vi "Single-Line To CSM Parts.vi"(11 "Single-line Text":string="asdfas @ * >> asdfas @ asvas ->    <register> //asdfas") -> (0 "Msg Type":T4, 1 "Comment Pos":i32, 2 "Comments":T3, 3 "Property":T1[](array[typedef]))   [LabVIEW 2017]
uses:
  Single-Line Type.ctl
  CSM Part Property.ctl
  Single-Line Selection Type.ctl
  <vilib>/regexp/Match Regular Expression.xnode
  _Shared/CSM Shared.lvlib
panel:
  out "Array":string[](array[string])=["status@asdfasf ", ">>", " abcdef@xaef ", "->", "<register>"]
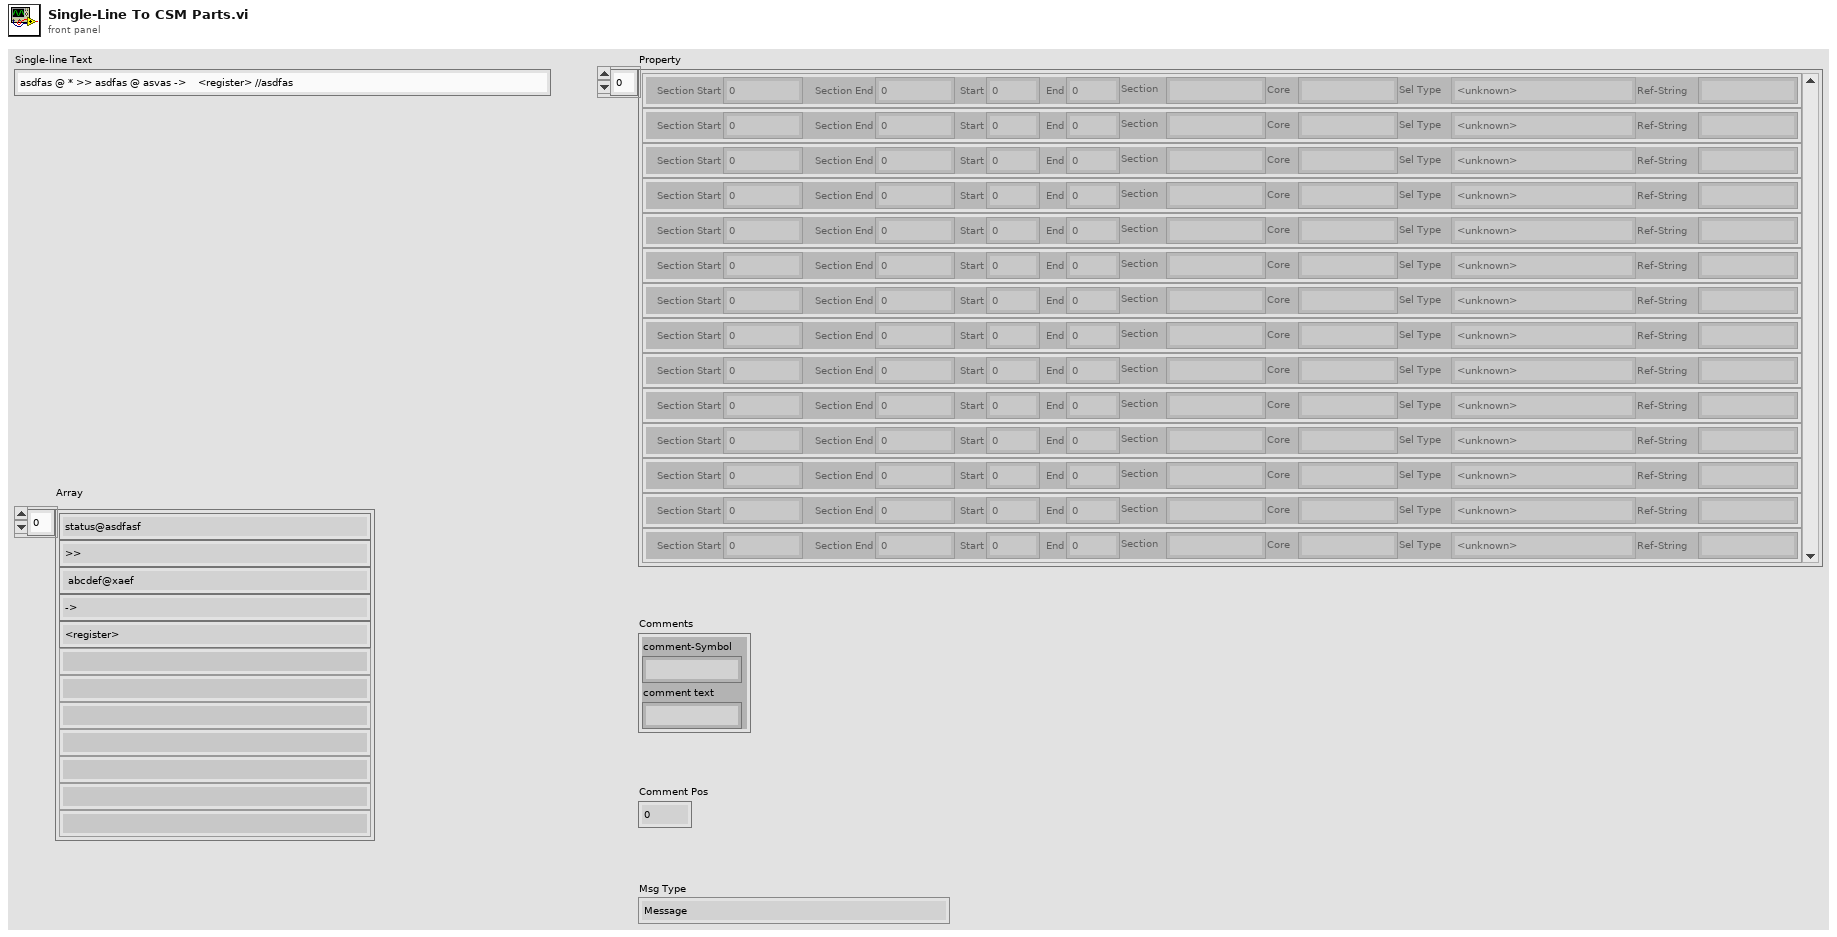
[diagram p1: front panel]
types:
  T1 = typedef "CSM Part Property.ctl" = cluster{"Section Start":u32, "Section End":u32, "Start":u32, "End":u32, "Section":string, "Core":string, "Sel Type":T2, "Ref-String":string}
  T2 = typedef "Single-Line Selection Type.ctl" = enum16{"<unknown>", "Reg-SourceSignal", "Reg-@Seperator", "Reg-ArgSymbol", "Reg-TargetAPI", "Reg-Module", "Reg-Symbol", "Reg-Oper", "Msg-State", "Msg-Arg", "Msg-ArgSymbol", "Msg-Symbol", "Msg-Module", "Broadcast-Signal", "Broadcast-ArgSymbol", "Broadcast-Arg", "Broadcast-Symbol", "Broadcast-Oper", "Comment-Symbol", "Comment-Content"}
  T3 = cluster{"comment-Symbol":string, "comment text":string}
  T4 = typedef "Single-Line Type.ctl" = enum16{"Message", "Broadcast", "Registration"}
  T5 = cluster{"Single-line Text":string, "Single-line Text":string}
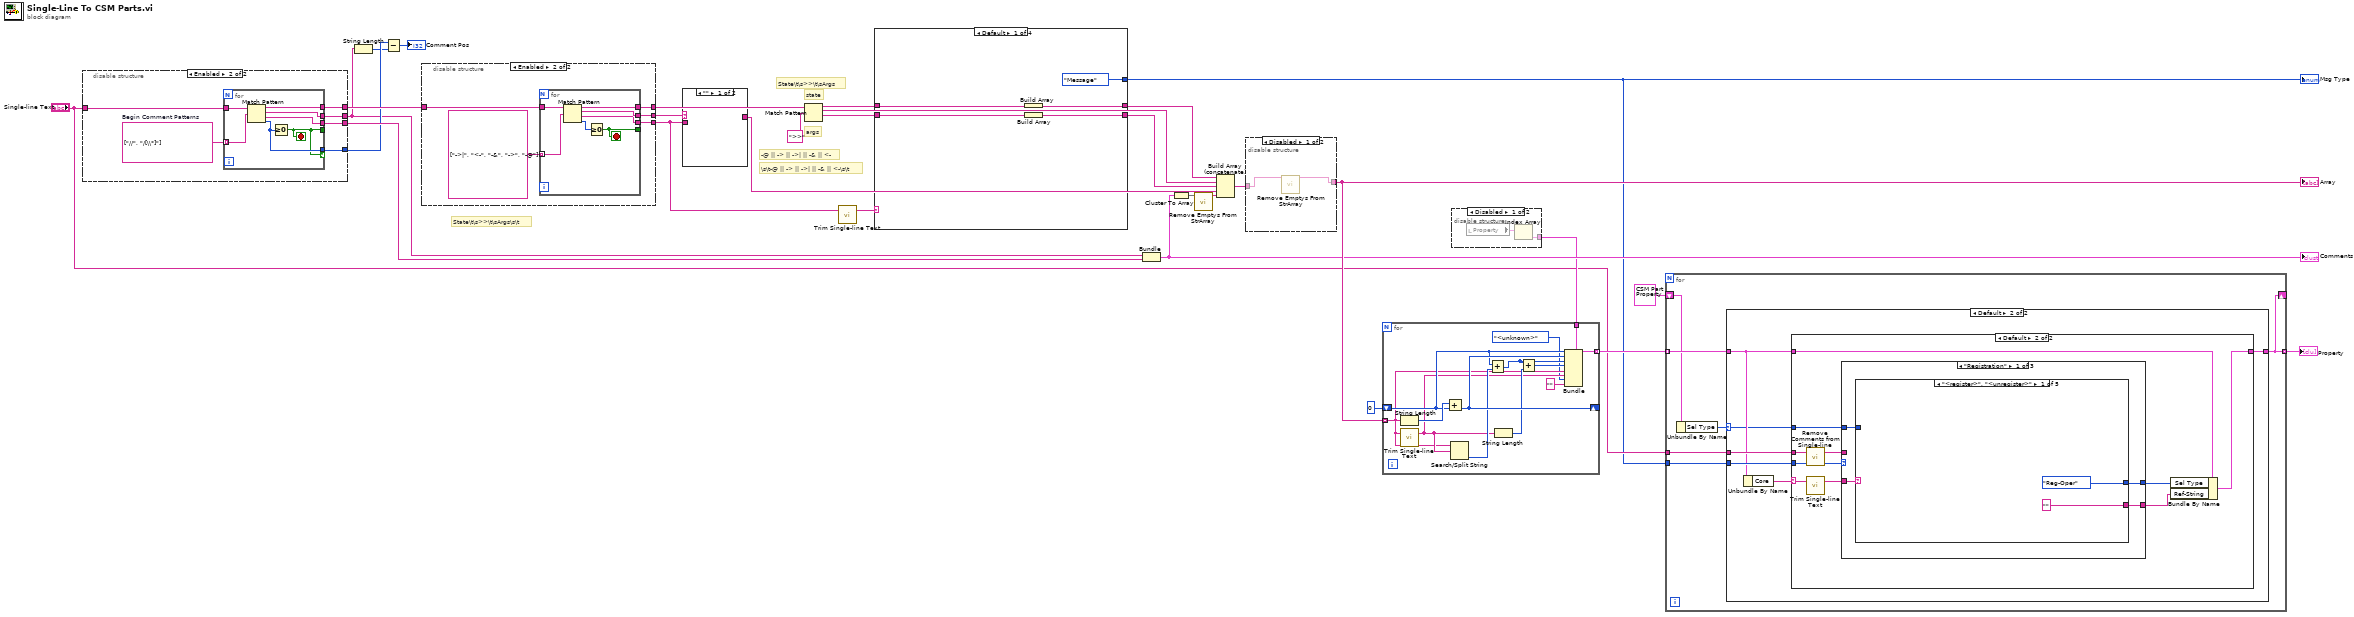
[diagram p0: block diagram]
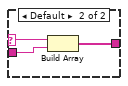
[diagram p2: hidden frame]
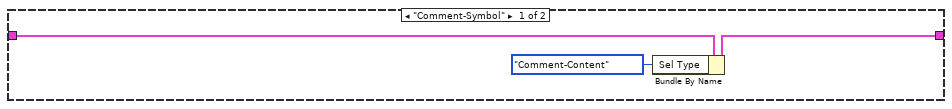
[diagram p5: hidden frame]
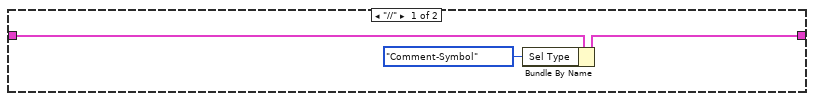
[diagram p6: hidden frame]
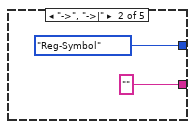
[diagram p7: hidden frame]
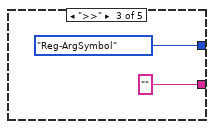
[diagram p8: hidden frame]
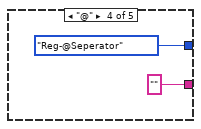
[diagram p9: hidden frame]
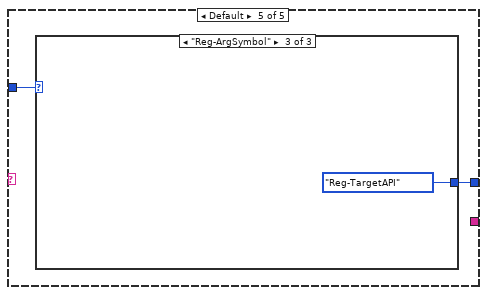
[diagram p10: hidden frame]
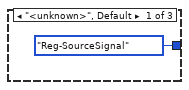
[diagram p11: hidden frame]
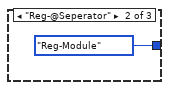
[diagram p12: hidden frame]
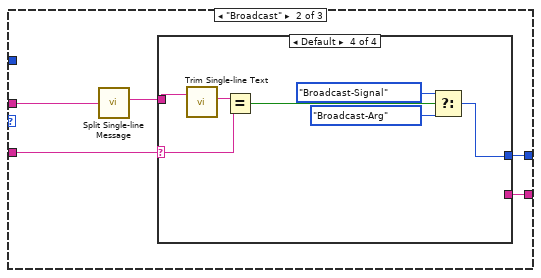
[diagram p13: hidden frame]
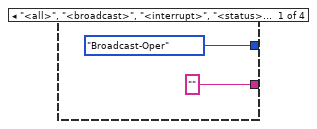
[diagram p14: hidden frame]
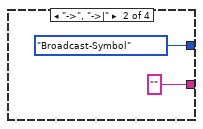
[diagram p15: hidden frame]
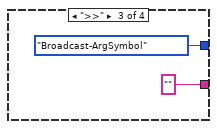
[diagram p16: hidden frame]
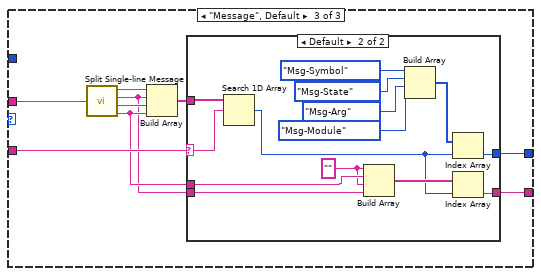
[diagram p17: hidden frame]
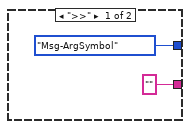
[diagram p18: hidden frame]
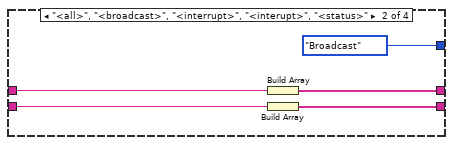
[diagram p19: hidden frame]
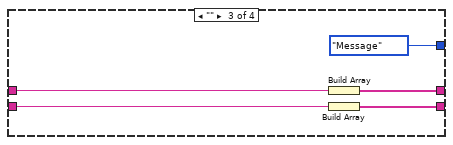
[diagram p20: hidden frame]
diagram:
  # "-@ || -> || ->| || -& || <-"
  # "\\s\\t-@ || -> || ->| || -& || <-\\s\\t"
  # "State\\t\\s>>\\t\\sArgs"
  # "State\\t\\s>>\\t\\sArgs\\s\\t"
  # "args"
  # "state"
  n1 = disable-structure shown="Enabled" {
    disable-tunnel: [w33 w153] -> w29
    disable-tunnel: [w32 w152] -> w13
    disable-tunnel: [w31 w151] -> w20
    disable-tunnel: "Single-line Text" -> [w30 w154]
    disable-tunnel: [_ w149] -> w15
    frame Disabled {
      n2 = xnode "Match Regular Expression"("input string"=w30, "regular expression"="[\\t\\s]*-@|->|<-|-&[\\t\\s]*") -> ("before match"=w33:string, "whole match"=w32:string, "after match"=w31:string)  [unwired: 4 in, 2 out]
    }
    frame Enabled {
      w150 = string[] ["//", "/[\\*]"]  # Begin Comment Patterns
      n3 = for {
        tunnel: w154 -> [w161]
        tunnel: w150 -> [w160] mode=indexing
        tunnel: [w155] -> _
        tunnel: [w159] -> w153
        tunnel: [w158] -> w152
        tunnel: [w157] -> w151
        tunnel: [w156] -> w149 if=w155
        stop <- w155 stop-if-true
        n4 = Match Pattern(string=w161, regular expression=w160) -> (before substring=w159:string, match substring=w158:string, after substring=w157:string, offset past match=w156:i32)  [unwired: 1 in]
        n5 = Greater Or Equal To 0?(x=w156) -> (x >= 0?=w155:bool)
      }
    }
  }
  n6 = String Length(string=w13) -> (length=w14:i32)
  n7 = Subtract(x=w15, y=w14) -> (x-y=→"Comment Pos":i32)
  n8 = disable-structure shown="Enabled" {
    disable-tunnel: [w165 w283] -> w28
    disable-tunnel: [w164 w282] -> w5
    disable-tunnel: [w163 w281] -> w3
    disable-tunnel: w29 -> [w162 w285]
    frame Disabled {
      n9 = xnode "Match Regular Expression"("input string"=w162, "regular expression"="[\\t\\s]*-@|->|<-|-&[\\t\\s]*") -> ("before match"=w165:string, "whole match"=w164:string, "after match"=w163:string)  [unwired: 4 in, 2 out]
    }
    frame Enabled {
      n10 = for {
        tunnel: w285 -> [w292]
        tunnel: string[] ["->|", "<-", "-&", "->", "-@"] -> [w291] mode=indexing
        tunnel: [w289] -> _
        tunnel: [w288] -> w283
        tunnel: [w287] -> w282
        tunnel: [w286] -> w281
        stop <- w289 stop-if-true
        n11 = Match Pattern(string=w292, regular expression=w291) -> (before substring=w288:string, match substring=w287:string, after substring=w286:string, offset past match=w290:i32)  [unwired: 1 in]
        n12 = Greater Or Equal To 0?(x=w290) -> (x >= 0?=w289:bool)
      }
    }
  }
  n13 = case shown="\"\"" w5 {
    selector: w5 -> [_ w295]
    tunnel: w3 -> [_ w294]
    tunnel: [_ w293] -> w4
    frame "" {
    }
    frame Default {
      n14 = Build Array(w295, w294) -> (w293:string[])
    }
  }
  n15 = Match Pattern(string=w28, regular expression=">>") -> (before substring=w23:string, match substring=w26:string, after substring=w25:string)  [unwired: 1 in, 1 out]
  n16 = call "Trim Single-line Text.vi"("single-line text"=w3) -> ("trimed text"=w21:string)  [unwired: 2 in]
  n17 = case shown="Default" w21 {
    tunnel: w25 -> [w299 w304 w309 w317]
    tunnel: [w298 w303 w308 w312] -> w24
    tunnel: w23 -> [w300 w305 w310 w324]
    tunnel: [w297 w302 w307 w311] -> w22
    tunnel: [Single-Line_Type."Message" ("Msg Type") Single-Line_Type."Broadcast" ("Msg Type") Single-Line_Type."Message" ("Msg Type") Single-Line_Type."Registration" ("Msg Type")] -> w8
    frame Default {
      n18 = Build Array(w300) -> (w297:string[])
      n19 = Build Array(w299) -> (w298:string[])
    }
    frame "<all>", "<broadcast>", "<interrupt>", "<interupt>", "<status>" {
      n20 = Build Array(w305) -> (w302:string[])
      n21 = Build Array(w304) -> (w303:string[])
    }
    frame "" {
      n22 = Build Array(w310) -> (w307:string[])
      n23 = Build Array(w309) -> (w308:string[])
    }
    frame "<register>", "<unregister>" {
      w315 = "@" ("regular expression")
      n24 = Match Pattern(string=w324, regular expression=w315) -> (before substring=w323:string, match substring=w322:string, after substring=w321:string)  [unwired: 1 in, 1 out]
      n25 = Match Pattern(string=w317, regular expression=w315) -> (before substring=w318:string, match substring=w319:string, after substring=w320:string)  [unwired: 1 in, 1 out]
      n26 = Build Array(w323, w322, w321) -> (w313:string[])
      n27 = Build Array(w318, w319, w320) -> (w314:string[])
      n28 = call "Remove Emptys From StrArray.vi"("Array In"=w313) -> ("Array Out"=w311:string[])  [unwired: 10 in]
      n29 = call "Remove Emptys From StrArray.vi"("Array In"=w314) -> ("Array Out"=w312:string[])  [unwired: 10 in]
    }
  }
  "Msg Type" <- w8
  n30 = Bundle("Single-line Text"=w13, "Single-line Text"=w20) -> (w16:T5)  [unwired: 1 in]
  "Comments" <- w16
  n31 = Cluster To Array(cluster=w16) -> (array=w2:string[])
  n32 = call "Remove Emptys From StrArray.vi"("Array In"=w2) -> ("Array Out"=w1:string[])  [unwired: 10 in]
  n33 = Build Array (concatenate)(w22, w26, w24, w4, w1) -> (w17:string[])
  n34 = disable-structure shown="Disabled" {
    disable-tunnel: [w326 w327] -> w18
    disable-tunnel: w17 -> [w325 w327]
    frame Disabled {
      n35 = call "Remove Emptys From StrArray.vi"("Array In"=w325) -> ("Array Out"=w326:string[])  [unwired: 10 in]
    }
    frame Enabled {
    }
  }
  "Array" <- w18
  n36 = disable-structure shown="Disabled" {
    disable-tunnel: [w328 _] -> w10
    frame Disabled {
      n37 = local read "Property"() -> (w329:T1[])
      n38 = Index Array(array=w329) -> (element=w328:T1)  [unwired: 1 in]
    }
    frame Enabled {
    }
  }
  n39 = for {
    tunnel: w18 -> [w333] mode=indexing
    shift-right: [w341] -> _
    shift-left: u32 0 -> [w339]
    tunnel: [w340] -> w11 mode=indexing
    tunnel: w10 -> [w330]
    n40 = String Length(string=w333) -> (length=w342:i32)
    n41 = call "Trim Single-line Text.vi"("single-line text"=w333) -> ("trimed text"=w334:string)  [unwired: 2 in]
    n42 = Add(x=w342, y=w339) -> (x+y=w341:u32)
    n43 = Search/Split String(string=w333, search string/char (-)=w334) -> (offset of match=w338:i32)  [unwired: 1 in, 2 out]
    n44 = Add(x=w339, y=w338) -> (x+y=w337:u32)
    n45 = String Length(string=w334) -> (length=w336:i32)
    n46 = Add(x=w337, y=w336) -> (x+y=w335:u32)
    n47 = Bundle(cluster=w330, "Section Start"=w339, "Section End"=w341, "Start"=w337, "End"=w335, "Section"=w333, "Core"=w334, "Sel Type"=Single-Line_Selection_Type."<unknown>", "Ref-String"="" ("regular expression")) -> (w340:T1)
  }
  n48 = for {
    tunnel: w11 -> [w346] mode=indexing
    tunnel: "Single-line Text" -> [w348]
    tunnel: w8 -> [w347]
    tunnel: [w343] -> w7 mode=indexing
    shift-right: [w343] -> _
    shift-left: T1 {"Section Start"=0, "Section End"=0, "Start"=0, "End"=0, "Section"="", "Core"="", "Sel Type"=enum."<unknown>", "Ref-String"=""} -> [w345]
    n49 = Unbundle By Name(w345) -> ("Sel Type"=w344:T2)
    n50 = case shown="Default" w344 {
      selector: w344 -> [_ w352]
      tunnel: w348 -> [_ w357]
      tunnel: w347 -> [_ w355]
      tunnel: [w350 w354] -> w343
      tunnel: w346 -> [w351 w353]
      frame "Comment-Symbol" {
        n51 = Bundle By Name(cluster=w351, "Sel Type"=Single-Line_Selection_Type."Comment-Content") -> (w350:T1)
      }
      frame Default {
        n52 = Unbundle By Name(w353) -> ("Core"=w356:string)
        n53 = case shown="Default" w356 {
          selector: w356 -> [_ w369]
          tunnel: w357 -> [_ w370]
          tunnel: w355 -> [_ w368]
          tunnel: w353 -> [w360 w365]
          tunnel: [w359 w362] -> w354
          tunnel: w352 -> [_ w361]
          frame "//" {
            n54 = Bundle By Name(cluster=w360, "Sel Type"=Single-Line_Selection_Type."Comment-Symbol") -> (w359:T1)
          }
          frame Default {
            n55 = call "Remove Comments from Single-line.vi"("single-line text"=w370) -> ("single-line text without comments"=w366:string)  [unwired: 2 in]
            n56 = call "Trim Single-line Text.vi"("single-line text"=w369) -> ("trimed text"=w367:string)  [unwired: 2 in]
            n57 = case shown="\"Registration\"" w368 {
              tunnel: w367 -> [w372 w392 w414]
              tunnel: [w374 w391 w413] -> w364
              tunnel: [w373 w390 w412] -> w363
              tunnel: w366 -> [_ w389 w411]
              tunnel: w361 -> [w371 _ _]
              frame "Registration" {
                n58 = case shown="\"<register>\", \"<unregister>\"" w372 {
                  tunnel: [Single-Line_Selection_Type."Reg-Oper" Single-Line_Selection_Type."Reg-Symbol" Single-Line_Selection_Type."Reg-ArgSymbol" Single-Line_Selection_Type."Reg-@Seperator" w383] -> w374
                  tunnel: ["" ("Ref-String") "" ("Ref-String") "" ("Ref-String") "" ("Ref-String") _] -> w373
                  tunnel: w371 -> [_ _ _ _ w384]
                  frame "<register>", "<unregister>" {
                  }
                  frame "->", "->|" {
                  }
                  frame ">>" {
                  }
                  frame "@" {
                  }
                  frame Default {
                    n59 = case shown="\"Reg-ArgSymbol\"" w384 {
                      tunnel: [Single-Line_Selection_Type."Reg-SourceSignal" ("Sel Type") Single-Line_Selection_Type."Reg-Module" ("Sel Type") Single-Line_Selection_Type."Reg-TargetAPI" ("Sel Type")] -> w383
                      frame "<unknown>", Default {
                      }
                      frame "Reg-@Seperator" {
                      }
                      frame "Reg-ArgSymbol" {
                      }
                    }
                  }
                }
              }
              frame "Broadcast" {
                n60 = call "Split Single-line Message.vi"("single-line text"=w389) -> ("state"=w388:string)  [unwired: 6 in, 3 out]
                n61 = case shown="Default" w392 {
                  selector: w392 -> [_ _ _ w404]
                  tunnel: [Single-Line_Selection_Type."Broadcast-Oper" Single-Line_Selection_Type."Broadcast-Symbol" Single-Line_Selection_Type."Broadcast-ArgSymbol" w399] -> w391
                  tunnel: ["" ("Ref-String") "" ("Ref-String") "" ("Ref-String") _] -> w390
                  tunnel: w388 -> [_ _ _ w405]
                  frame "<all>", "<broadcast>", "<interrupt>", "<status>" {
                  }
                  frame "->", "->|" {
                  }
                  frame ">>" {
                  }
                  frame Default {
                    n62 = call "Trim Single-line Text.vi"("single-line text"=w405) -> ("trimed text"=w403:string)  [unwired: 2 in]
                    n63 = Equal?(x=w403, y=w404) -> (x = y?=w402:bool)
                    n64 = Select(t=Single-Line_Selection_Type."Broadcast-Signal", s=w402, f=Single-Line_Selection_Type."Broadcast-Arg") -> (s? t:f=w399:T2)
                  }
                }
              }
              frame "Message", Default {
                n65 = call "Split Single-line Message.vi"("single-line text"=w411) -> ("operator"=w410:string, "state"=w406:string, "args"=w409:string, "source/target"=w407:string)  [unwired: 6 in]
                n66 = Build Array(w410, w406, w409, w407) -> (w408:string[])
                n67 = case shown="Default" w414 {
                  selector: w414 -> [_ w429]
                  tunnel: [Single-Line_Selection_Type."Msg-ArgSymbol" w424] -> w413
                  tunnel: ["" ("Ref-String") w422] -> w412
                  tunnel: w408 -> [_ w430]
                  tunnel: w407 -> [_ w419]
                  tunnel: w406 -> [_ w418]
                  frame ">>" {
                  }
                  frame Default {
                    w417 = "" ("element")
                    n68 = Search 1D Array(1D array=w430, element=w429) -> (index of element=w420:i32)  [unwired: 1 in]
                    n69 = Build Array(w417, w419, w417, w418) -> (w421:string[])
                    n70 = Build Array(Single-Line_Selection_Type."Msg-Symbol", Single-Line_Selection_Type."Msg-State", Single-Line_Selection_Type."Msg-Arg", Single-Line_Selection_Type."Msg-Module") -> (w423:T2[])
                    n71 = Index Array(array=w423, index=w420) -> (element=w424:T2)
                    n72 = Index Array(array=w421, index=w420) -> (element=w422:string)
                  }
                }
              }
            }
            n73 = Bundle By Name(cluster=w365, "Sel Type"=w364, "Ref-String"=w363) -> (w362:T1)
          }
        }
      }
    }
  }
  "Property" <- w7
